vi "Sound player.vi"() -> ()   [LabVIEW 2014]
uses:
  winmm.dll
panel:
  in  "경로":path
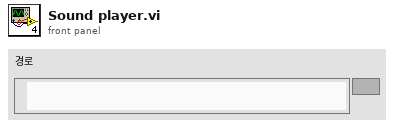
[diagram p1: front panel]
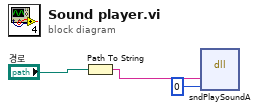
[diagram p0: block diagram]
diagram:
  n1 = Path To String(path="경로") -> (string=w2:string)
  n2 = dll-call lib="winmm.dll" fn="sndPlaySoundA"("SoundFile"=w2, "Options"=u32 0) -> ()  [unwired: 6 in, 2 out]
